vi "media_mobile.vi"(1 "Campioni media mobile":i32, 2 "Waveform in":waveform(dbl)) -> (0 "Waveform out":waveform(dbl))   [LabVIEW 2012]
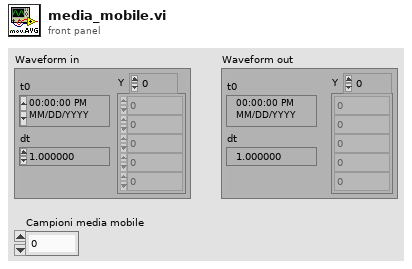
[diagram p1: front panel]
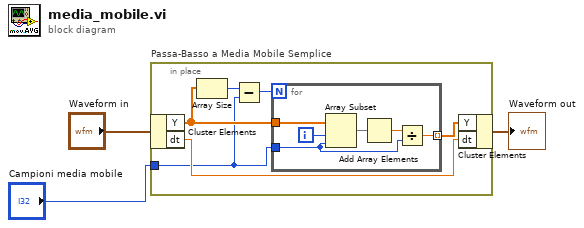
[diagram p0: block diagram]
diagram:
  n1 = in-place "Passa-Basso a Media Mobile Semplice" {
    in-place-border: "Campioni media mobile" -> [w5]
    n2 = in-place-cluster #1("Waveform in") -> ("Y"=w7:dbl[], "dt"=w6:dbl)
    n3 = Array Size(array=w7) -> (size(s)=w9:i32)
    n4 = Subtract(x=w9, y=w5) -> (x-y=w8:i32)
    n5 = for {
      N: w8 -> [_]
      tunnel: w7 -> [w15]
      tunnel: w5 -> [w10]
      tunnel: [w11] -> w4 mode=indexing
      i -> [w14]
      n6 = Array Subset(array=w15, index=w14, length=w10) -> (w13:dbl[])
      n7 = Add Array Elements(numeric array=w13) -> (sum=w12:dbl)
      n8 = Divide(x=w12, y=w10) -> (x/y=w11:dbl)
    }
    n9 = in-place-cluster #1("Y"=w4, "dt"=w6) -> (→"Waveform out":waveform(dbl))
  }
